vi "Demultiplexer.vi"() -> ()   [LabVIEW 2020]
panel:
  in  "DATA D":bool
  out "Y3":bool
  out "Y2":bool
  out "Y1":bool
  out "Y0":bool
  in  "B":bool
  in  "A":bool
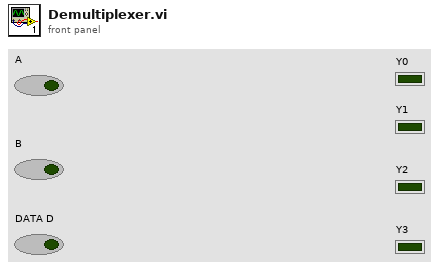
[diagram p1: front panel]
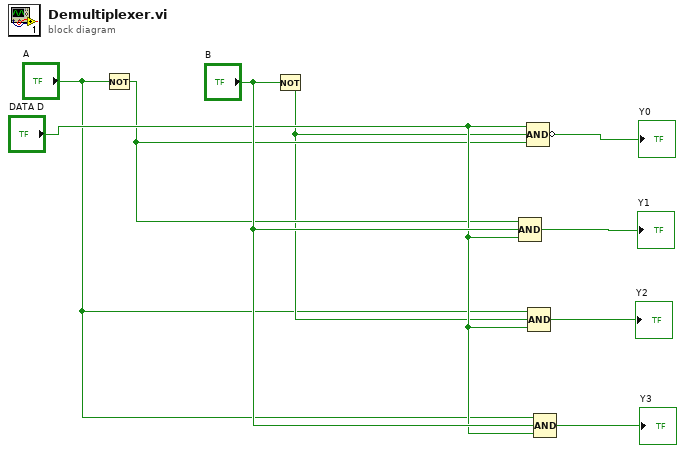
[diagram p0: block diagram]
diagram:
  n1 = Not(x="A") -> (.not. x?=w5:bool)
  n2 = Not(x="B") -> (.not. x?=w2:bool)
  n3 = Compound Arithmetic op=AND(w5, "B", "DATA D") -> (→"Y1":bool)
  n4 = Compound Arithmetic op=AND("DATA D", w2, w5) -> (invert →"Y0":bool)
  n5 = Compound Arithmetic op=AND("A", w2, "DATA D") -> (→"Y2":bool)
  n6 = Compound Arithmetic op=AND("A", "B", "DATA D") -> (→"Y3":bool)
